vi "Create Transfer.vi"(7 "id":i32, 8 "error in (no error)":errorcluster, 10 "name":string, 11 "Buffers":refnum<class "Buffers.lvclass">) -> (0 "error out":errorcluster, 3 "Transfer out":refnum<class "Transfer.lvclass">)   [LabVIEW 2021, in "DSF Core.lvlib" / "Transfer.lvclass"]
uses:
  Transfer.lvclass
  Buffers/Buffers.lvclass
  Transfer.lvclass/Transfer.ctl
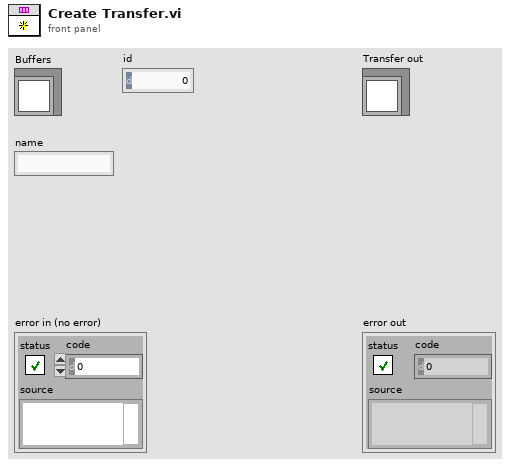
[diagram p1: front panel]
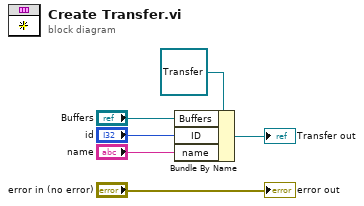
[diagram p0: block diagram]
diagram:
  n1 = Bundle By Name(cluster=refnum<class "Transfer.lvclass"> refnum ("Transfer in"), "Buffers"="Buffers", "ID"="id", "name"="name") -> (→"Transfer out":refnum<class "Transfer.lvclass">)
  "error out" <- "error in (no error)"
